vi "check stop runtime.vi"(11 "Commands":T1) -> (3 "stop?":bool)   [LabVIEW 2013, in "Standard Engine Runtime.lvclass"]
uses:
  Standard Engine Runtime.lvclass
  Commands.ctl
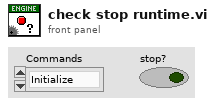
[diagram p1: front panel]
types:
  T1 = typedef "Standard Engine Runtime.lvclass/Commands.ctl" = enum16{"Initialize", "Start", "Pause", "Safe State", "Normal", "Stop", "Shutdown"}
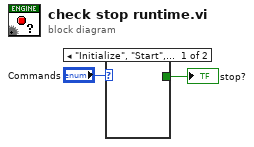
[diagram p0: block diagram]
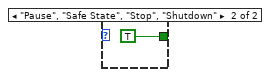
[diagram p2: hidden frame]
diagram:
  n1 = case shown="\"Initialize\", \"Start\", \"Normal\"" "Commands" {
    tunnel: [_ TRUE] -> w1
    frame "Initialize", "Start", "Normal" {
    }
    frame "Pause", "Safe State", "Stop", "Shutdown" {
    }
  }
  "stop?" <- w1
